vi "Cluster_to_CipheredString.vi"(0 "Usuario":string, 2 "password to cipher users":string, 3 "BitKeyType(256)":u16, 5 "Actions":string, 7 "Account type":T1, 9 "Time Stamp":timestamp, 11 "error in (no error)":errorcluster) -> (8 "CypheredText":string, 15 "error out":errorcluster)   [LabVIEW 2012]
uses:
  typedef/User Accounts.ctl
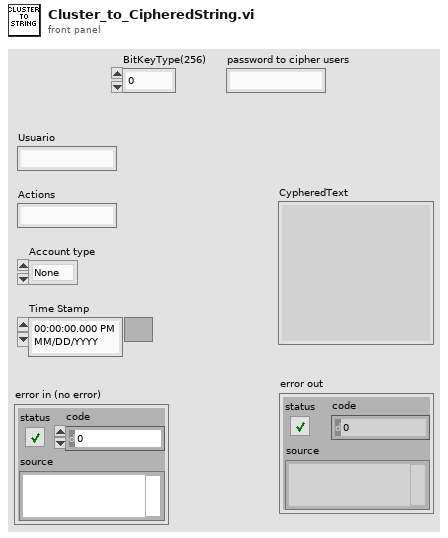
[diagram p1: front panel]
types:
  T1 = typedef "User Accounts.ctl" = enum16{"None", "User", "Admin"}
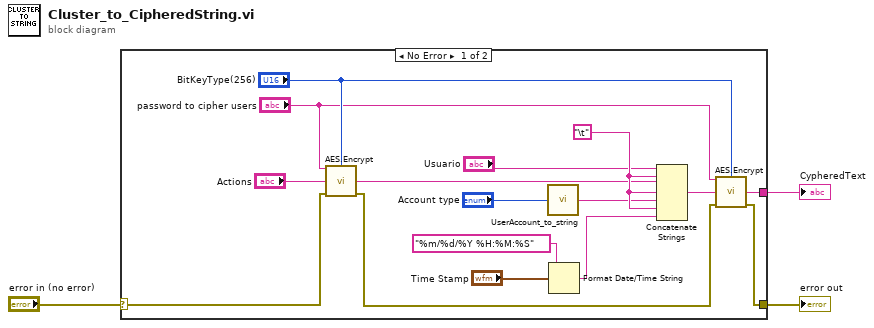
[diagram p0: block diagram]
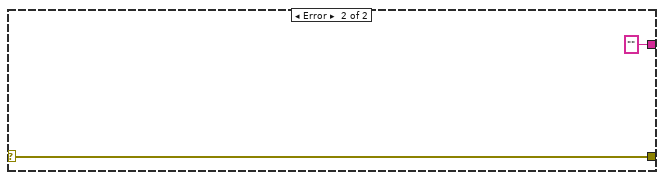
[diagram p2: hidden frame]
diagram:
  n1 = case shown="No Error" "error in (no error)" {
    selector: "error in (no error)" -> [w8 w21]
    tunnel: [w6 w21] -> w2
    tunnel: [w11 "" ("CypheredText")] -> w1
    frame No Error {
      w18 = "\t"
      n2 = call <vilib>:"AES.Encrypt.vi"("Password"="password to cipher users", "BitKeyType (256)"="BitKeyType(256)", "PlainText"="Actions", "error in"=w8) -> ("CypheredText"=w9:string, "error out"=w7:errorcluster)  [unwired: 10 in]
      n3 = call "UserAccount_to_string.vi"("Account"="Account type") -> ("String"=w17:string)
      n4 = Format Date/Time String(time format string (%c)="%m/%d/%Y %H:%M:%S" ("format string"), seconds (now)="Time Stamp") -> (date/time string=w15:string)  [unwired: 1 in]
      n5 = Concatenate Strings("Usuario", w18, w9, w18, w17, w18, w15) -> (w19:string)
      n6 = call <vilib>:"AES.Encrypt.vi"("Password"="password to cipher users", "BitKeyType (256)"="BitKeyType(256)", "PlainText"=w19, "error in"=w7) -> ("CypheredText"=w11:string, "error out"=w6:errorcluster)  [unwired: 10 in]
    }
    frame Error {
    }
  }
  "error out" <- w2
  "CypheredText" <- w1
